vi "MoveAbs.vi"(8 "error in (no error)":errorcluster, 11 "DMC 3600 in":refnum<class "DMC 3600.lvclass">) -> (0 "error out":errorcluster, 3 "DMC 3600 out":refnum<class "DMC 3600.lvclass">)   [LabVIEW 2019, in "DMC 3600.lvclass"]
uses:
  DMC 3600.lvclass
  LLB/Commonly VI/Main Glb.vi
  LLB/Commonly VI.lvlib
  LLB/DMC3600/LTDMC.lvlib
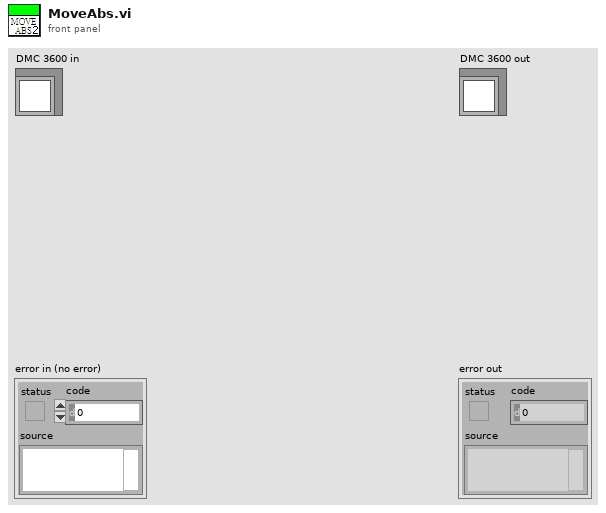
[diagram p1: front panel]
types:
  T1 = cluster{"AxisName":string, "Accel":dbl, "Deaccel":dbl, "Speed":dbl, "Sramp":dbl}[]
  T2 = cluster{"AxisName":string, "Accel":dbl, "Deaccel":dbl, "Speed":dbl, "Sramp":dbl}
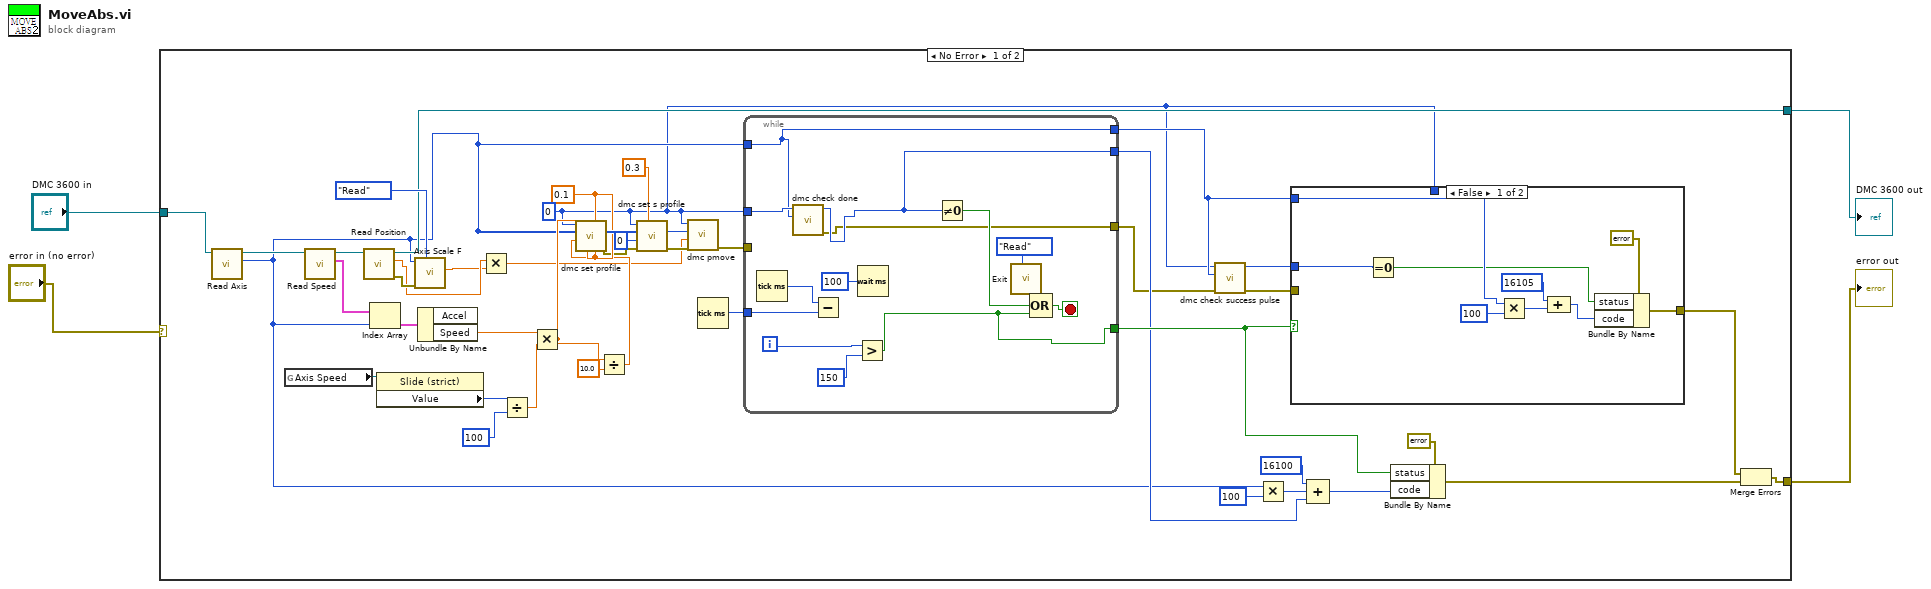
[diagram p0: block diagram]
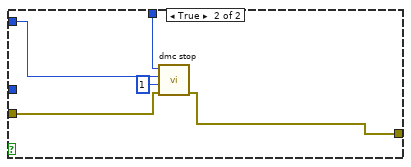
[diagram p2: hidden frame]
diagram:
  n1 = case shown="No Error" "error in (no error)" {
    selector: "error in (no error)" -> [_ w75]
    tunnel: "DMC 3600 in" -> [w24 w76]
    tunnel: [w23 w76] -> w2
    tunnel: [w6 w75] -> w1
    frame No Error {
      w20 = 0.1 ("Tdec")
      w9 = u16 0 ("posi_mode")
      n2 = call-dynamic "Read Axis.vi"("AxisCard in"=w24) -> ("Axis"=w21:u32, "AxisCard out"=w46:refnum<class "DMC 3600.lvclass">)  [unwired: 8 in, 1 out]
      n3 = global read "Main Glb.vi" "Axis Speed"() -> (w33:refnum<vi>)
      n4 = call-dynamic "Read Speed.vi"("AxisCard in"=w46) -> ("AxisSpeed"=w45:T1, "AxisCard out"=w35:refnum<class "DMC 3600.lvclass">)  [unwired: 8 in, 1 out]
      n5 = call-dynamic "Read Position.vi"("AxisCard in"=w35) -> ("error out"=w28:errorcluster, "Position"=w27:dbl, "AxisCard out"=w23:refnum<class "DMC 3600.lvclass">)  [unwired: 8 in]
      n6 = Index Array(array=w45, index=w21) -> (element=w44:T2)
      n7 = property class="Slide (strict)"(reference=w33) -> ("Value"=w32:i32)  [unwired: 1 in, 2 out]
      n8 = call "Axis Scale F.vi"("Enum"=enum16{"Initial", "Read"}."Read", "error In"=w28, "Axis"=w21) -> ("Scale"=w26:dbl)  [unwired: 7 in, 1 out]
      n9 = Unbundle By Name(w44) -> ("Speed"=w30:dbl)  [unwired: 1 out]
      n10 = Multiply(x=w27, y=w26) -> (x*y=w14:dbl)
      n11 = Divide(x=w32, y=100) -> (x/y=w29:dbl)
      n12 = Multiply(x=w30, y=w29) -> (x*y=w22:dbl)
      n13 = Divide(x=w22, y=10.0) -> (x/y=w19:dbl)
      n14 = call "dmc set profile.vi"("stop_vel"=w19, "Tdec"=w20, "Tacc"=w20, "Max_Vel"=w22, "Min_Vel"=w19, "axis"=w21, "CardNo"=w9) -> ("error out"=w18:errorcluster)  [unwired: 3 in, 1 out]
      n15 = call "dmc set s profile.vi"("s_para"=0.3, "error in (no error)"=w18, "s_mode"=u16 0, "axis"=w21, "CardNo"=w9) -> ("error out"=w17:errorcluster)  [unwired: 5 in, 1 out]
      n16 = call "dmc pmove.vi"("error in (no error)"=w17, "dist"=w14, "axis"=w21, "CardNo"=w9) -> ("error out"=w13:errorcluster)  [unwired: 6 in, 1 out]
      n17 = Tick Count (ms)() -> (millisecond timer value=w43:u32)
      n18 = while {
        tunnel: w21 -> [w64]
        tunnel: w43 -> [w72]
        tunnel: [w64] -> w12
        tunnel: [w61] -> w37
        tunnel: [w63] -> w36
        tunnel: w13 -> [_]
        tunnel: w9 -> [w65]
        tunnel: [w62] -> w11
        i -> [w69]
        stop <- w70 stop-if-true
        n19 = Tick Count (ms)() -> (millisecond timer value=w73:u32)
        n20 = call "dmc check done.vi"("axis"=w64, "CardNo"=w65) -> ("error out"=w62:errorcluster, "function return"=w63:i16)  [unwired: 8 in]
        n21 = Subtract(x=w73, y=w72) -> ()  [unwired: 1 out]
        n22 = Greater?(x=w69, y=u32 150) -> (0:w61:bool)
        n23 = Wait (ms)(milliseconds to wait=u32 100) -> ()  [unwired: 1 out]
        n24 = Not Equal To 0?(x=w63) -> (x != 0?=w66:bool)
        n25 = call "Exit.vi"("Enum"=enum16{"Initial", "Read", "Write"}."Read") -> ("ExitOut"=w68:bool)  [unwired: 10 in]
        n26 = Compound Arithmetic op=OR(w68, w66, w61) -> (w70:bool)
      }
      n27 = call "dmc check success pulse.vi"("error in (no error)"=w11, "axis"=w12, "CardNo"=w9) -> ("error out"=w8:errorcluster, "function return"=w7:i16)  [unwired: 7 in]
      n28 = Multiply(x=w21, y=u32 100) -> (x*y=w41:u32)
      n29 = case shown="False" w37 {
        tunnel: w12 -> [w51 w60]
        tunnel: w9 -> [_ w59]
        tunnel: w8 -> [_ w57]
        tunnel: w7 -> [w55 _]
        tunnel: [w47 w56] -> w5
        frame False {
          n30 = Equal To 0?(x=w55) -> (x = 0?=w48:bool)
          n31 = Multiply(x=w51, y=u32 100) -> (x*y=w53:u32)
          n32 = Compound Arithmetic op=ADD(16105, w53) -> (w49:u32)
          n33 = Bundle By Name(cluster=errorcluster {"status"=FALSE, "code"=0, "source"=""} ("error constant"), "status"=w48, "code"=w49) -> (w47:errorcluster)
        }
        frame True {
          n34 = call "dmc stop.vi"("error in (no error)"=w57, "stop_mode"=u16 1, "axis"=w60, "CardNo"=w59) -> ("error out"=w56:errorcluster)  [unwired: 6 in, 1 out]
        }
      }
      n35 = Compound Arithmetic op=ADD(16100, w41, w36) -> (w38:u32)
      n36 = Bundle By Name(cluster=errorcluster {"status"=FALSE, "code"=0, "source"=""} ("error constant"), "status"=w37, "code"=w38) -> (w10:errorcluster)
      n37 = Merge Errors(w5, w10) -> (w6:errorcluster)
    }
    frame Error {
    }
  }
  "error out" <- w1
  "DMC 3600 out" <- w2
